vi "Martinas Aging Program v1.0c.vi"() -> ()   [LabVIEW 2011]
uses:
  <vilib>/ULx/Create Channel.llb/ULx Create Channel (DO-Digital Output).vi
  <vilib>/ULx/Write.llb/ULx Write (Digital U32 1Chan 1Samp).vi
  <instrlib>/Keithley 24XX/Keithley 24XX.lvlib
panel:
  out "Numeric":dbl
  out "Cell Settings Array":T1(array[cluster])=[{"Measure?"=TRUE, "Area (cm^2)"=0.0, "Cell Label"="", "Cell Description"="", "Time between scans (min)"=0.0, "Cell Position"=1, "Scan settings in queue"=0, "Sample holder"=1.0}, {"Measure?"=TRUE, "Area (cm^2)"=0.0, "Cell Label"="", "Cell Description"="", "Time between scans (min)"=0.0, "Cell Position"=2, "Scan settings in queue"=0, "Sample holder"=1.0}, {"Measure?"=TRUE, "Area (cm^2)"=0.0, "Cell Label"="", "Cell Description"="", "Time between scans (min)"=0.0, "Cell Position"=3, "Scan settings in queue"=0, "Sample holder"=1.0}, {"Measure?"=TRUE, "Area (cm^2)"=0.0, "Cell Label"="", "Cell Description"="", "Time between scans (min)"=0.0, "Cell Position"=4, "Scan settings in queue"=0, "Sample holder"=1.0}, {"Measure?"=TRUE, "Area (cm^2)"=0.0, "Cell Label"="", "Cell Description"="", "Time between scans (min)"=0.0, "Cell Position"=5, "Scan settings in queue"=0, "Sample holder"=1.0}, {"Measure?"=TRUE, "Area (cm^2)"=0.0, "Cell Label"="", "Cell Description"="", "Time between scans (min)"=0.0, "Cell Position"=6, "Scan settings in queue"=0, "Sample holder"=1.0}, {"Measure?"=TRUE, "Area (cm^2)"=0.0, "Cell Label"="", "Cell Description"="", "Time between scans (min)"=0.0, "Cell Position"=7, "Scan settings in queue"=0, "Sample holder"=1.0}, {"Measure?"=TRUE, "Area (cm^2)"=0.0, "Cell Label"="", "Cell Description"="", "Time between scans (min)"=0.0, "Cell Position"=8, "Scan settings in queue"=0, "Sample holder"=1.0}, {"Measure?"=TRUE, "Area (cm^2)"=0.0, "Cell Label"="", "Cell Description"="", "Time between scans (min)"=0.0, "Cell Position"=9, "Scan settings in queue"=0, "Sample holder"=1.0}, {"Measure?"=TRUE, "Area (cm^2)"=0.0, "Cell Label"="", "Cell Description"="", "Time between scans (min)"=0.0, "Cell Position"=10, "Scan settings in queue"=0, "Sample holder"=1.0}, {"Measure?"=TRUE, "Area (cm^2)"=0.0, "Cell Label"="", "Cell Description"="", "Time between scans (min)"=0.0, "Cell Position"=11, "Scan settings in queue"=0, "Sample holder"=1.0}, {"Measure?"=TRUE, "Area (cm^2)"=0.0, "Cell Label"="", "Cell Description"="", "Time between scans (min)"=0.0, "Cell Position"=12, "Scan settings in queue"=0, "Sample holder"=1.0}, {"Measure?"=TRUE, "Area (cm^2)"=0.0, "Cell Label"="", "Cell Description"="", "Time between scans (min)"=0.0, "Cell Position"=13, "Scan settings in queue"=0, "Sample holder"=1.0}, {"Measure?"=TRUE, "Area (cm^2)"=0.0, "Cell Label"="", "Cell Description"="", "Time between scans (min)"=0.0, "Cell Position"=14, "Scan settings in queue"=0, "Sample holder"=1.0}, {"Measure?"=TRUE, "Area (cm^2)"=0.0, "Cell Label"="", "Cell Description"="", "Time between scans (min)"=0.0, "Cell Position"=15, "Scan settings in queue"=0, "Sample holder"=1.0}, {"Measure?"=TRUE, "Area (cm^2)"=0.0, "Cell Label"="", "Cell Description"="", "Time between scans (min)"=0.0, "Cell Position"=16, "Scan settings in queue"=0, "Sample holder"=1.0}] {"Scan settings in queue" items=["Regular", "Inverted"]}
  in  "Port":refnum<k21>="Dev0/AuxPort"
  in  "VISA resource name":refnum<visa-resource-name>="GPIB0::24::INSTR"
  in  "Tab Control":T2(tab)
  in  "Cell Settings Array 1":T3(array[cluster])=[{"Measure?"=TRUE, "Area (cm^2)"=0.0, "Cell Label"="", "Cell Description"="", "Time between scans (s)"=0.0, "Cell Position"=1, "Scan settings in queue"=0, "Sample holder"=1.0}, {"Measure?"=TRUE, "Area (cm^2)"=0.0, "Cell Label"="", "Cell Description"="", "Time between scans (s)"=0.0, "Cell Position"=2, "Scan settings in queue"=0, "Sample holder"=1.0}, {"Measure?"=TRUE, "Area (cm^2)"=0.0, "Cell Label"="", "Cell Description"="", "Time between scans (s)"=0.0, "Cell Position"=3, "Scan settings in queue"=0, "Sample holder"=1.0}, {"Measure?"=TRUE, "Area (cm^2)"=0.0, "Cell Label"="", "Cell Description"="", "Time between scans (s)"=0.0, "Cell Position"=4, "Scan settings in queue"=0, "Sample holder"=1.0}, {"Measure?"=TRUE, "Area (cm^2)"=0.0, "Cell Label"="", "Cell Description"="", "Time between scans (s)"=0.0, "Cell Position"=5, "Scan settings in queue"=0, "Sample holder"=1.0}, {"Measure?"=TRUE, "Area (cm^2)"=0.0, "Cell Label"="", "Cell Description"="", "Time between scans (s)"=0.0, "Cell Position"=6, "Scan settings in queue"=0, "Sample holder"=1.0}, {"Measure?"=TRUE, "Area (cm^2)"=0.0, "Cell Label"="", "Cell Description"="", "Time between scans (s)"=0.0, "Cell Position"=7, "Scan settings in queue"=0, "Sample holder"=1.0}, {"Measure?"=TRUE, "Area (cm^2)"=0.0, "Cell Label"="", "Cell Description"="", "Time between scans (s)"=0.0, "Cell Position"=8, "Scan settings in queue"=0, "Sample holder"=1.0}, {"Measure?"=TRUE, "Area (cm^2)"=0.0, "Cell Label"="", "Cell Description"="", "Time between scans (s)"=0.0, "Cell Position"=9, "Scan settings in queue"=0, "Sample holder"=1.0}, {"Measure?"=TRUE, "Area (cm^2)"=0.0, "Cell Label"="", "Cell Description"="", "Time between scans (s)"=0.0, "Cell Position"=10, "Scan settings in queue"=0, "Sample holder"=1.0}, {"Measure?"=TRUE, "Area (cm^2)"=0.0, "Cell Label"="", "Cell Description"="", "Time between scans (s)"=0.0, "Cell Position"=11, "Scan settings in queue"=0, "Sample holder"=1.0}, {"Measure?"=TRUE, "Area (cm^2)"=0.0, "Cell Label"="", "Cell Description"="", "Time between scans (s)"=0.0, "Cell Position"=12, "Scan settings in queue"=0, "Sample holder"=1.0}, {"Measure?"=TRUE, "Area (cm^2)"=0.0, "Cell Label"="", "Cell Description"="", "Time between scans (s)"=0.0, "Cell Position"=13, "Scan settings in queue"=0, "Sample holder"=1.0}, {"Measure?"=TRUE, "Area (cm^2)"=0.0, "Cell Label"="", "Cell Description"="", "Time between scans (s)"=0.0, "Cell Position"=14, "Scan settings in queue"=0, "Sample holder"=1.0}, {"Measure?"=TRUE, "Area (cm^2)"=0.0, "Cell Label"="", "Cell Description"="", "Time between scans (s)"=0.0, "Cell Position"=15, "Scan settings in queue"=0, "Sample holder"=1.0}, {"Measure?"=TRUE, "Area (cm^2)"=0.0, "Cell Label"="", "Cell Description"="", "Time between scans (s)"=0.0, "Cell Position"=16, "Scan settings in queue"=0, "Sample holder"=1.0}] {"Scan settings in queue" items=["Regular", "Inverted", "Test"]}
  in  "Upload from Spreadsheet?":bool
  in  "Upload Spreadsheet path":path
  in  "Save to Spreadsheet?":bool
  in  "Save Spreadsheet Path":path
  in  "Cell Settings Array 2":T1(array[cluster])=[{"Measure?"=TRUE, "Area (cm^2)"=0.0, "Cell Label"="", "Cell Description"="", "Time between scans (min)"=0.0, "Cell Position"=1, "Scan settings in queue"=0, "Sample holder"=2.0}, {"Measure?"=TRUE, "Area (cm^2)"=0.0, "Cell Label"="", "Cell Description"="", "Time between scans (min)"=0.0, "Cell Position"=2, "Scan settings in queue"=0, "Sample holder"=2.0}, {"Measure?"=TRUE, "Area (cm^2)"=0.0, "Cell Label"="", "Cell Description"="", "Time between scans (min)"=0.0, "Cell Position"=3, "Scan settings in queue"=0, "Sample holder"=2.0}, {"Measure?"=TRUE, "Area (cm^2)"=0.0, "Cell Label"="", "Cell Description"="", "Time between scans (min)"=0.0, "Cell Position"=4, "Scan settings in queue"=0, "Sample holder"=2.0}, {"Measure?"=TRUE, "Area (cm^2)"=0.0, "Cell Label"="", "Cell Description"="", "Time between scans (min)"=0.0, "Cell Position"=5, "Scan settings in queue"=0, "Sample holder"=2.0}, {"Measure?"=TRUE, "Area (cm^2)"=0.0, "Cell Label"="", "Cell Description"="", "Time between scans (min)"=0.0, "Cell Position"=6, "Scan settings in queue"=0, "Sample holder"=2.0}, {"Measure?"=TRUE, "Area (cm^2)"=0.0, "Cell Label"="", "Cell Description"="", "Time between scans (min)"=0.0, "Cell Position"=7, "Scan settings in queue"=0, "Sample holder"=2.0}, {"Measure?"=TRUE, "Area (cm^2)"=0.0, "Cell Label"="", "Cell Description"="", "Time between scans (min)"=0.0, "Cell Position"=8, "Scan settings in queue"=0, "Sample holder"=2.0}, {"Measure?"=TRUE, "Area (cm^2)"=0.0, "Cell Label"="", "Cell Description"="", "Time between scans (min)"=0.0, "Cell Position"=9, "Scan settings in queue"=0, "Sample holder"=2.0}, {"Measure?"=TRUE, "Area (cm^2)"=0.0, "Cell Label"="", "Cell Description"="", "Time between scans (min)"=0.0, "Cell Position"=10, "Scan settings in queue"=0, "Sample holder"=2.0}, {"Measure?"=TRUE, "Area (cm^2)"=0.0, "Cell Label"="", "Cell Description"="", "Time between scans (min)"=0.0, "Cell Position"=11, "Scan settings in queue"=0, "Sample holder"=2.0}, {"Measure?"=TRUE, "Area (cm^2)"=0.0, "Cell Label"="", "Cell Description"="", "Time between scans (min)"=0.0, "Cell Position"=12, "Scan settings in queue"=0, "Sample holder"=2.0}, {"Measure?"=TRUE, "Area (cm^2)"=0.0, "Cell Label"="", "Cell Description"="", "Time between scans (min)"=0.0, "Cell Position"=13, "Scan settings in queue"=0, "Sample holder"=2.0}, {"Measure?"=TRUE, "Area (cm^2)"=0.0, "Cell Label"="", "Cell Description"="", "Time between scans (min)"=0.0, "Cell Position"=14, "Scan settings in queue"=0, "Sample holder"=2.0}, {"Measure?"=TRUE, "Area (cm^2)"=0.0, "Cell Label"="", "Cell Description"="", "Time between scans (min)"=0.0, "Cell Position"=15, "Scan settings in queue"=0, "Sample holder"=2.0}, {"Measure?"=TRUE, "Area (cm^2)"=0.0, "Cell Label"="", "Cell Description"="", "Time between scans (min)"=0.0, "Cell Position"=16, "Scan settings in queue"=0, "Sample holder"=2.0}] {"Scan settings in queue" items=["Regular", "Inverted", "Test"]}
  in  "Upload Spreadsheet path 2":path
  in  "Upload from Spreadsheet? 2":bool
  in  "Save Spreadsheet Path 2":path
  in  "Save to Spreadsheet?  2":bool
  in  "Cell Settings Array 3":T1(array[cluster])=[{"Measure?"=TRUE, "Area (cm^2)"=0.0, "Cell Label"="", "Cell Description"="", "Time between scans (min)"=0.0, "Cell Position"=1, "Scan settings in queue"=0, "Sample holder"=3.0}, {"Measure?"=TRUE, "Area (cm^2)"=0.0, "Cell Label"="", "Cell Description"="", "Time between scans (min)"=0.0, "Cell Position"=2, "Scan settings in queue"=0, "Sample holder"=3.0}, {"Measure?"=TRUE, "Area (cm^2)"=0.0, "Cell Label"="", "Cell Description"="", "Time between scans (min)"=0.0, "Cell Position"=3, "Scan settings in queue"=0, "Sample holder"=3.0}, {"Measure?"=TRUE, "Area (cm^2)"=0.0, "Cell Label"="", "Cell Description"="", "Time between scans (min)"=0.0, "Cell Position"=4, "Scan settings in queue"=0, "Sample holder"=3.0}, {"Measure?"=TRUE, "Area (cm^2)"=0.0, "Cell Label"="", "Cell Description"="", "Time between scans (min)"=0.0, "Cell Position"=5, "Scan settings in queue"=0, "Sample holder"=3.0}, {"Measure?"=TRUE, "Area (cm^2)"=0.0, "Cell Label"="", "Cell Description"="", "Time between scans (min)"=0.0, "Cell Position"=6, "Scan settings in queue"=0, "Sample holder"=3.0}, {"Measure?"=TRUE, "Area (cm^2)"=0.0, "Cell Label"="", "Cell Description"="", "Time between scans (min)"=0.0, "Cell Position"=7, "Scan settings in queue"=0, "Sample holder"=3.0}, {"Measure?"=TRUE, "Area (cm^2)"=0.0, "Cell Label"="", "Cell Description"="", "Time between scans (min)"=0.0, "Cell Position"=8, "Scan settings in queue"=0, "Sample holder"=3.0}, {"Measure?"=TRUE, "Area (cm^2)"=0.0, "Cell Label"="", "Cell Description"="", "Time between scans (min)"=0.0, "Cell Position"=9, "Scan settings in queue"=0, "Sample holder"=3.0}, {"Measure?"=TRUE, "Area (cm^2)"=0.0, "Cell Label"="", "Cell Description"="", "Time between scans (min)"=0.0, "Cell Position"=10, "Scan settings in queue"=0, "Sample holder"=3.0}, {"Measure?"=TRUE, "Area (cm^2)"=0.0, "Cell Label"="", "Cell Description"="", "Time between scans (min)"=0.0, "Cell Position"=11, "Scan settings in queue"=0, "Sample holder"=3.0}, {"Measure?"=TRUE, "Area (cm^2)"=0.0, "Cell Label"="", "Cell Description"="", "Time between scans (min)"=0.0, "Cell Position"=12, "Scan settings in queue"=0, "Sample holder"=3.0}, {"Measure?"=TRUE, "Area (cm^2)"=0.0, "Cell Label"="", "Cell Description"="", "Time between scans (min)"=0.0, "Cell Position"=13, "Scan settings in queue"=0, "Sample holder"=3.0}, {"Measure?"=TRUE, "Area (cm^2)"=0.0, "Cell Label"="", "Cell Description"="", "Time between scans (min)"=0.0, "Cell Position"=14, "Scan settings in queue"=0, "Sample holder"=3.0}, {"Measure?"=TRUE, "Area (cm^2)"=0.0, "Cell Label"="", "Cell Description"="", "Time between scans (min)"=0.0, "Cell Position"=15, "Scan settings in queue"=0, "Sample holder"=3.0}, {"Measure?"=TRUE, "Area (cm^2)"=0.0, "Cell Label"="", "Cell Description"="", "Time between scans (min)"=0.0, "Cell Position"=16, "Scan settings in queue"=0, "Sample holder"=3.0}] {"Scan settings in queue" items=["Regular", "Inverted", "Test"]}
  in  "Upload Spreadsheet path 3":path
  in  "Upload from Spreadsheet? 3":bool
  in  "Save Spreadsheet Path 3":path
  in  "Save to Spreadsheet?  3":bool
  in  "Cell Settings Array 4":T1(array[cluster])=[{"Measure?"=TRUE, "Area (cm^2)"=0.0, "Cell Label"="", "Cell Description"="", "Time between scans (min)"=0.0, "Cell Position"=1, "Scan settings in queue"=0, "Sample holder"=4.0}, {"Measure?"=TRUE, "Area (cm^2)"=0.0, "Cell Label"="", "Cell Description"="", "Time between scans (min)"=0.0, "Cell Position"=2, "Scan settings in queue"=0, "Sample holder"=4.0}, {"Measure?"=TRUE, "Area (cm^2)"=0.0, "Cell Label"="", "Cell Description"="", "Time between scans (min)"=0.0, "Cell Position"=3, "Scan settings in queue"=0, "Sample holder"=4.0}, {"Measure?"=TRUE, "Area (cm^2)"=0.0, "Cell Label"="", "Cell Description"="", "Time between scans (min)"=0.0, "Cell Position"=4, "Scan settings in queue"=0, "Sample holder"=4.0}, {"Measure?"=TRUE, "Area (cm^2)"=0.0, "Cell Label"="", "Cell Description"="", "Time between scans (min)"=0.0, "Cell Position"=5, "Scan settings in queue"=0, "Sample holder"=4.0}, {"Measure?"=TRUE, "Area (cm^2)"=0.0, "Cell Label"="", "Cell Description"="", "Time between scans (min)"=0.0, "Cell Position"=6, "Scan settings in queue"=0, "Sample holder"=4.0}, {"Measure?"=TRUE, "Area (cm^2)"=0.0, "Cell Label"="", "Cell Description"="", "Time between scans (min)"=0.0, "Cell Position"=7, "Scan settings in queue"=0, "Sample holder"=4.0}, {"Measure?"=TRUE, "Area (cm^2)"=0.0, "Cell Label"="", "Cell Description"="", "Time between scans (min)"=0.0, "Cell Position"=8, "Scan settings in queue"=0, "Sample holder"=4.0}, {"Measure?"=TRUE, "Area (cm^2)"=0.0, "Cell Label"="", "Cell Description"="", "Time between scans (min)"=0.0, "Cell Position"=9, "Scan settings in queue"=0, "Sample holder"=4.0}, {"Measure?"=TRUE, "Area (cm^2)"=0.0, "Cell Label"="", "Cell Description"="", "Time between scans (min)"=0.0, "Cell Position"=10, "Scan settings in queue"=0, "Sample holder"=4.0}, {"Measure?"=TRUE, "Area (cm^2)"=0.0, "Cell Label"="", "Cell Description"="", "Time between scans (min)"=0.0, "Cell Position"=11, "Scan settings in queue"=0, "Sample holder"=4.0}, {"Measure?"=TRUE, "Area (cm^2)"=0.0, "Cell Label"="", "Cell Description"="", "Time between scans (min)"=0.0, "Cell Position"=12, "Scan settings in queue"=0, "Sample holder"=4.0}, {"Measure?"=TRUE, "Area (cm^2)"=0.0, "Cell Label"="", "Cell Description"="", "Time between scans (min)"=0.0, "Cell Position"=13, "Scan settings in queue"=0, "Sample holder"=4.0}, {"Measure?"=TRUE, "Area (cm^2)"=0.0, "Cell Label"="", "Cell Description"="", "Time between scans (min)"=0.0, "Cell Position"=14, "Scan settings in queue"=0, "Sample holder"=4.0}, {"Measure?"=TRUE, "Area (cm^2)"=0.0, "Cell Label"="", "Cell Description"="", "Time between scans (min)"=0.0, "Cell Position"=15, "Scan settings in queue"=0, "Sample holder"=4.0}, {"Measure?"=TRUE, "Area (cm^2)"=0.0, "Cell Label"="", "Cell Description"="", "Time between scans (min)"=0.0, "Cell Position"=16, "Scan settings in queue"=0, "Sample holder"=4.0}] {"Scan settings in queue" items=["Regular", "Inverted", "Test"]}
  in  "Upload Spreadsheet path 4":path
  in  "Upload from Spreadsheet? 4":bool
  in  "Save Spreadsheet Path 4":path
  in  "Save to Spreadsheet?  4":bool
  in  "Stop Scan":bool
  in  "Start Scan":bool
  out "Table":string[][](table)
  out "JV Curve":cluster{"Y":dbl[], "Y":dbl[]}[](graph)
  in  "Upload to the Queue":bool
  in  "Stop Labview":bool
  in  "Scan settings":u16(ring) items=["Regular", "Inverted", "Test"]
  in  "Scan Settings JV":T4={"Light Intensity (Suns)"=1.0, "Stabilization Time (s)"=5.0, "Maximum Voltage (V)"=0.0, "Minimum Voltage (V)"=-1.0, "Range Options"=0, "Scan Direction\nDU (T), UD (F)"=TRUE, "Step Size (V)"=0.01, "Source Delay (s)"=0.15} {"Range Options" items=["Auto Range", "Semi-Auto Range", "100 uA", "1 mA", "10 mA", "100 mA", "1A"]}
  in  "Scan Setting Name":string
  in  "Add to Menu ring":bool
  out "Show me Scan \nSettings JV set":T4={"Light Intensity (Suns)"=1.0, "Stabilization Time (s)"=5.0, "Maximum Voltage (V)"=0.0, "Minimum Voltage (V)"=-1.0, "Range Options"=0, "Scan Direction\nDU (T), UD (F)"=TRUE, "Step Size (V)"=0.01, "Source Delay (s)"=0.15} {"Range Options" items=["Auto Range", "Semi-Auto Range", "100 uA", "1 mA", "10 mA", "100 mA", "1A"]}
  in  "Delete from Menu Ring":bool
  in  "Queue":T5(array[cluster]) {"Scan settings in queue" items=["Regular", "Inverted", "Test"]; "Time of the last scan (s)" format="%<%H:%M:%S>t"; "When did you stick it in?" format="%<%H:%M:%S>t"; "Time to next scan (s)" format="%<%H:%M:%S>t"; "Time in rig (s)" format="%<%H:%M:%S>t"}
  out "TIMER":dbl format="%<%H:%M:%S>t"
  out "Username":string caption="Logged in as:"
  # "Cell Ageing Routine"
  # "Time between Scans (s)"
  # "Cell\nPosition"
  # "Sample\nHolder"
  # "On = working cell\nOff = not working cell"
  # "Area"
  # "Label"
  # "Comment"
  # "Scan Settings"
  # "Time between Scans (s)"
  # "Cell\nPosition"
  # "Sample\nHolder"
  # "On = working cell\nOff = not working cell"
  # "Area"
  # "Label"
  # "Comment"
  # "Scan Settings"
  # "Time between Scans (s)"
  # "Cell\nPosition"
  # "Sample\nHolder"
  # "On = working cell\nOff = not working cell"
  # "Area"
  # "Label"
  # "Comment"
  # "Scan Settings"
  # "Time between Scans (s)"
  # "Cell\nPosition"
  # "Sample\nHolder"
  # "On = working cell\nOff = not working cell"
  # "Area"
  # "Label"
  # "Comment"
  # "Scan Settings"
  # "Area\n(cm^2)"
  # "Scan\nwait(s)"
  # "Cell \nposition"
  # "Time in rig\n(hrs)"
  # "Time since last scan (hrs)"
  # "Scan\nnumber"
  # "Time\nZero"
  # "Time of \nlast scan"
  # "Sample\nHolder"
  # "On = working\nOff = not working"
  # "Label"
  # "Comment"
  # "Scan Settings"
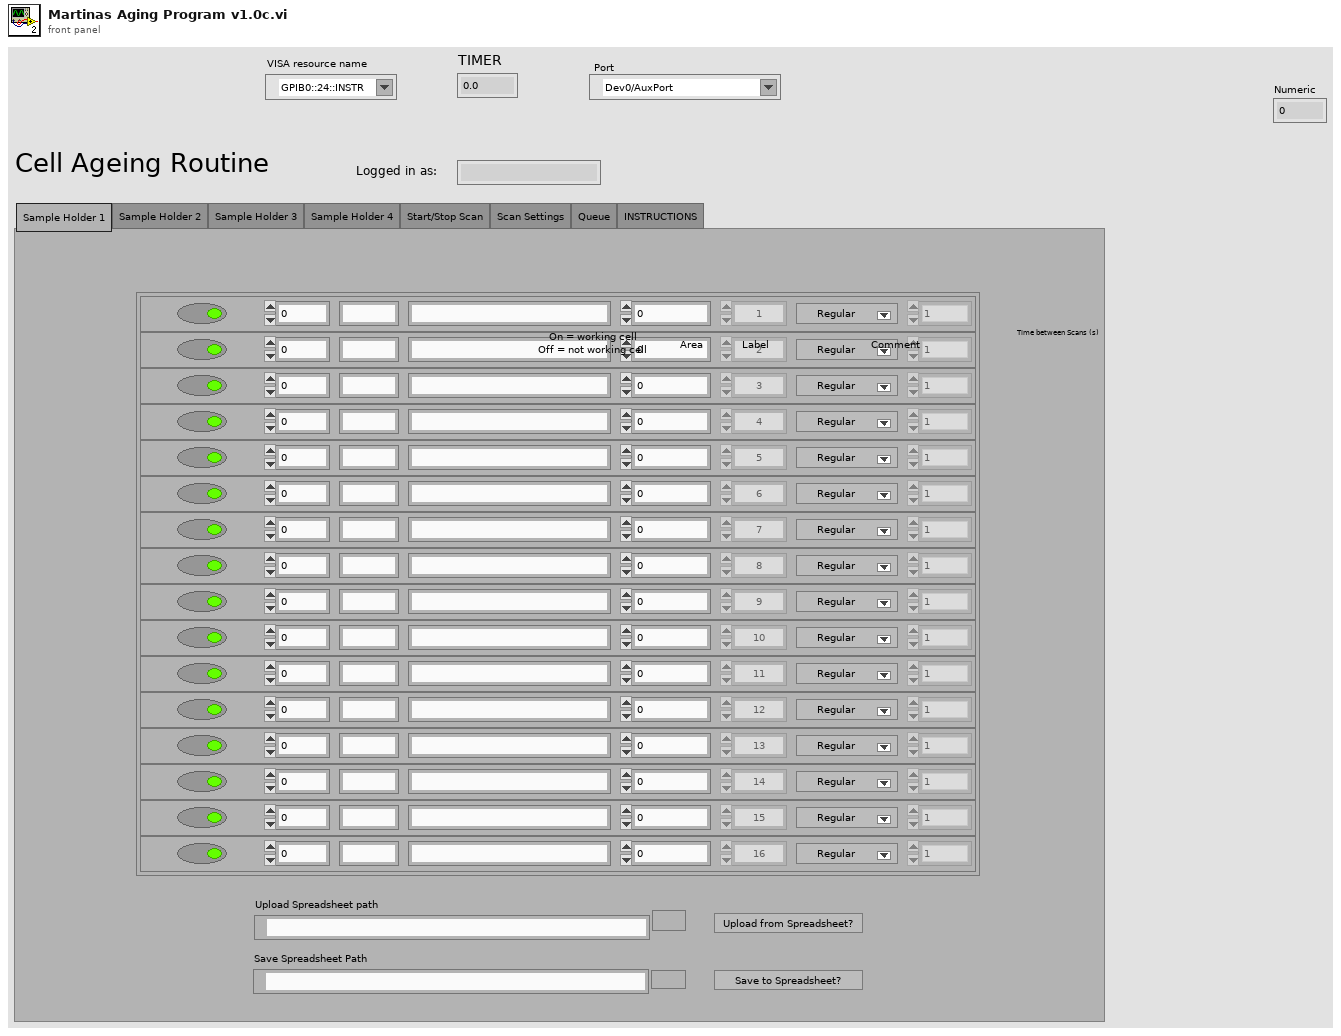
[diagram p1: front panel]
types:
  T1 = cluster{"Measure?":bool, "Area (cm^2)":dbl, "Cell Label":string, "Cell Description":string, "Time between scans (min)":dbl, "Cell Position":i32, "Scan settings in queue":u16, "Sample holder":dbl}[]
  T2 = enum32{"Sample Holder 1", "Sample Holder 2", "Sample Holder 3", "Sample Holder 4", "Start/Stop Scan", "Scan Settings", "Queue", "INSTRUCTIONS"}
  T3 = cluster{"Measure?":bool, "Area (cm^2)":dbl, "Cell Label":string, "Cell Description":string, "Time between scans (s)":dbl, "Cell Position":i32, "Scan settings in queue":u16, "Sample holder":dbl}[]
  T4 = cluster{"Light Intensity (Suns)":dbl, "Stabilization Time (s)":dbl, "Maximum Voltage (V)":dbl, "Minimum Voltage (V)":dbl, "Range Options":u16, "Scan Direction\nDU (T), UD (F)":bool, "Step Size (V)":dbl, "Source Delay (s)":dbl}
  T5 = cluster{"Measure?":bool, "Area (cm^2)":dbl, "Cell Label":string, "Cell Description":string, "Cell Position":i32, "Time in rig (s)":dbl, "Time to next scan (s)":dbl, "Scan number":dbl, "When did you stick it in?":dbl, "Time between scans (s)":dbl, "Time of the last scan (s)":dbl, "Scan settings in queue":u16, "Sample Holder":dbl}[]
  T6 = enum8{"Enabled", "Disabled", "Disabled and Grayed Out"}
  T7 = cluster{"Light Intensity (Suns)":dbl, "Stabilization Time (s)":dbl, "Maximum Voltage (V)":dbl, "Minimum Voltage (V)":dbl, "Range Options":u16, "Scan Direction\nDU (T), UD (F)":bool, "Step Size (V)":dbl, "Source Delay (s)":dbl}[]
  T8 = cluster{"Measure?":bool, "Area (cm^2)":dbl, "Cell Label":string, "Cell Description":string, "Cell Position":i32, "Time in rig (s)":dbl, "Time to next scan (s)":dbl, "Scan number":dbl, "When did you stick it in?":dbl, "Time between scans (s)":dbl, "Time of the last scan (s)":dbl, "Scan settings in queue":u16, "Sample Holder":dbl}
  T9 = typedef "imagedata.ctl" = cluster{"image type":i32, "image depth":i32, "image":u8[], "mask":u8[], "colors":u32[], "Rectangle":cluster{"left":i16, "top":i16, "right":i16, "bottom":i16}}
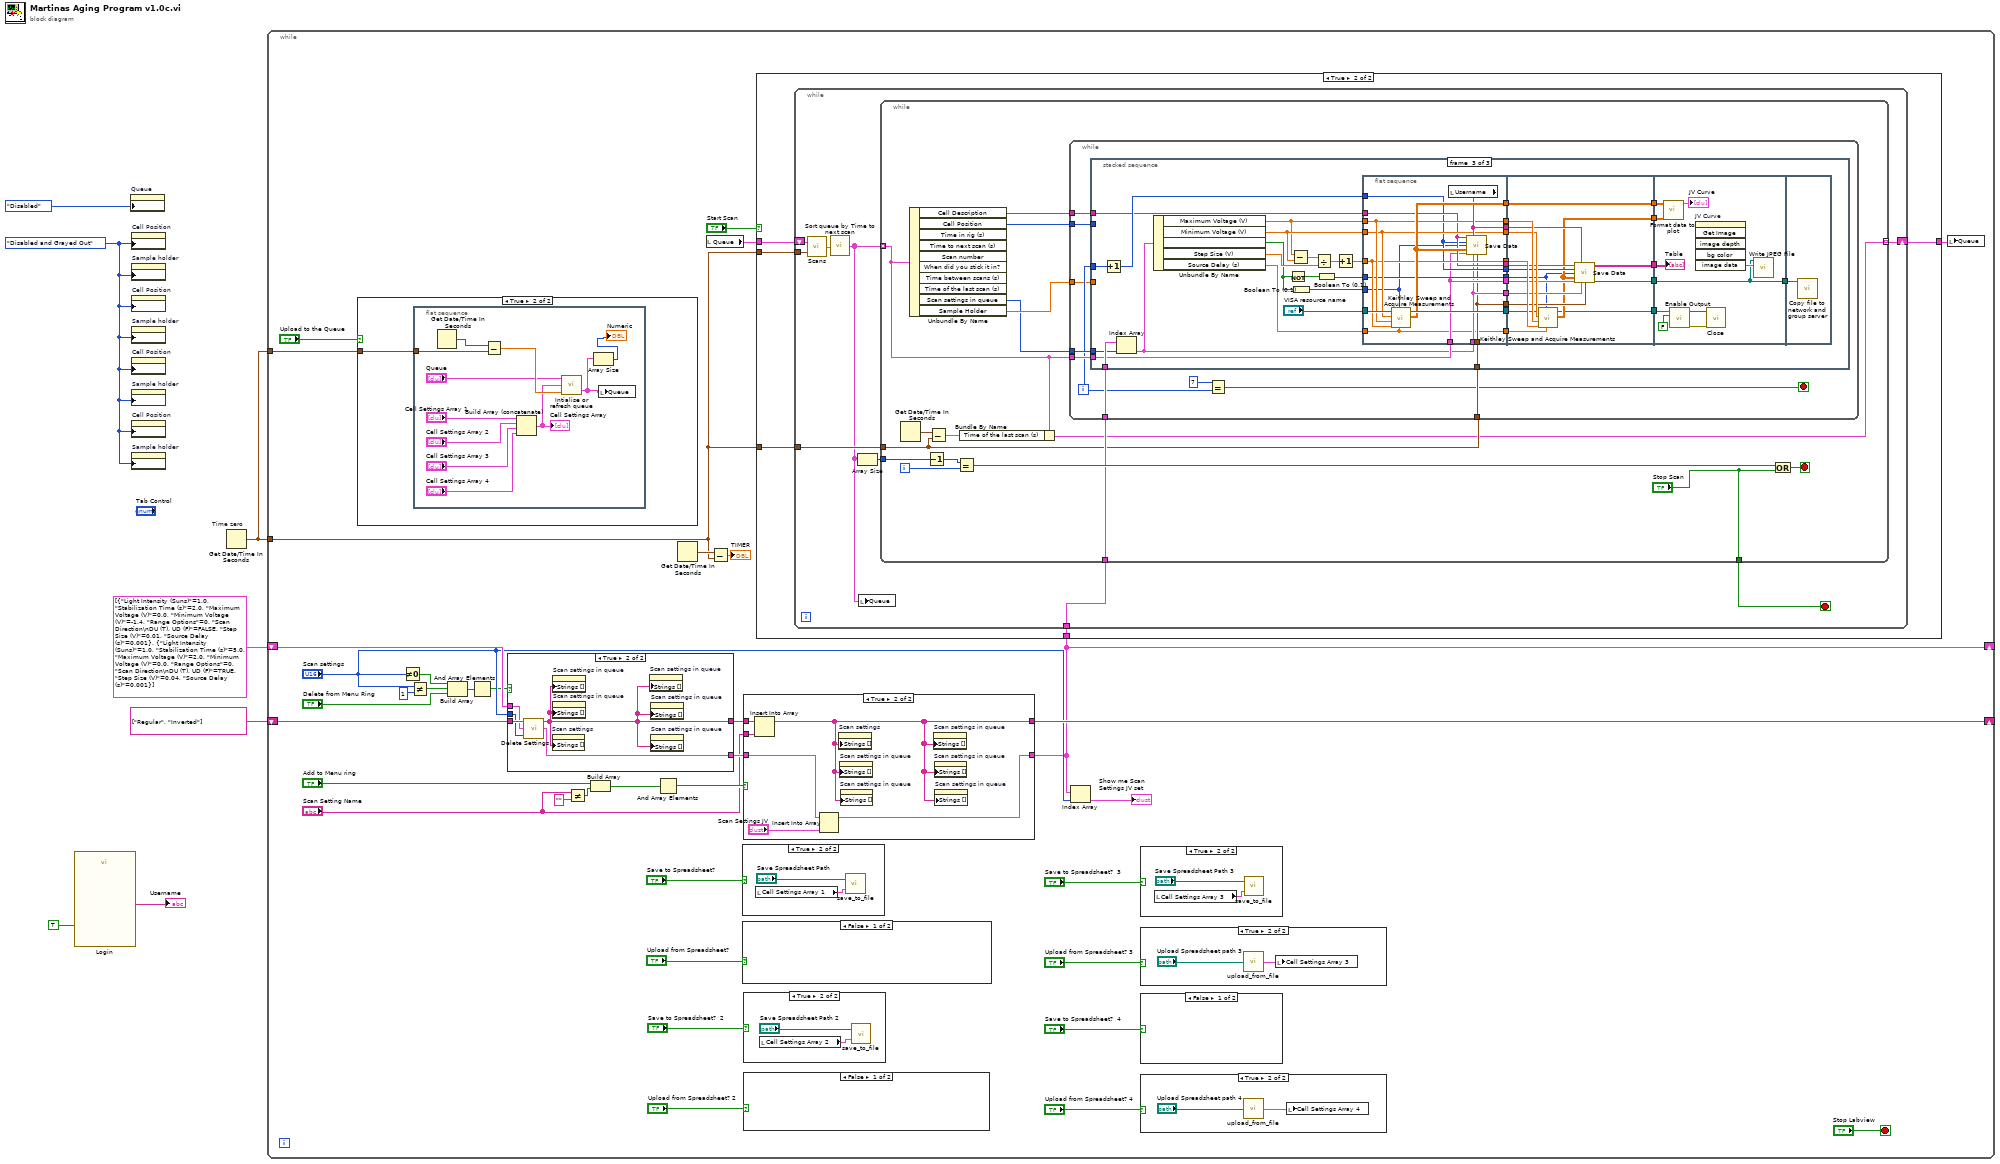
[diagram p0: block diagram]
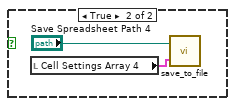
[diagram p2: hidden frame]
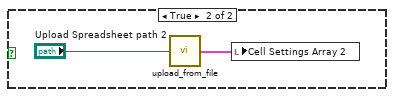
[diagram p7: hidden frame]
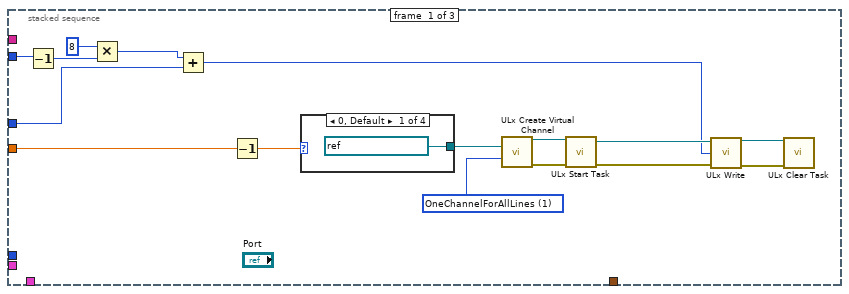
[diagram p9: hidden frame]
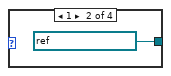
[diagram p10: hidden frame]
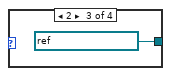
[diagram p11: hidden frame]
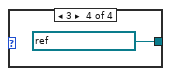
[diagram p12: hidden frame]
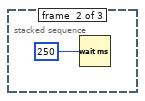
[diagram p13: hidden frame]
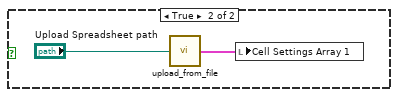
[diagram p18: hidden frame]
diagram:
  w4 = T6."Disabled and Grayed Out" ("Disabled")
  n1 = call "Login"("Enable"=TRUE) -> ("Username"=→"Username":string)  [unwired: 16 in, 2 out]
  n2 = property on="Queue" class="Arr (strict)"("DisabledEnum"=T6."Disabled" ("Disabled")) -> ()  [unwired: 2 in, 2 out]
  n3 = property on="Cell Position" class="DigNum (strict)"("DisabledEnum"=w4) -> ()  [unwired: 2 in, 2 out]
  n4 = property on="Sample holder" class="DigNum (strict)"("DisabledEnum"=w4) -> ()  [unwired: 2 in, 2 out]
  n5 = property on="Cell Position" class="DigNum (strict)"("DisabledEnum"=w4) -> ()  [unwired: 2 in, 2 out]
  n6 = property on="Sample holder" class="DigNum (strict)"("DisabledEnum"=w4) -> ()  [unwired: 2 in, 2 out]
  n7 = property on="Cell Position" class="DigNum (strict)"("DisabledEnum"=w4) -> ()  [unwired: 2 in, 2 out]
  n8 = property on="Sample holder" class="DigNum (strict)"("DisabledEnum"=w4) -> ()  [unwired: 2 in, 2 out]
  n9 = property on="Cell Position" class="DigNum (strict)"("DisabledEnum"=w4) -> ()  [unwired: 2 in, 2 out]
  n10 = property on="Sample holder" class="DigNum (strict)"("DisabledEnum"=w4) -> ()  [unwired: 2 in, 2 out]
  n11 = Get Date/Time In Seconds "Time zero"() -> (seconds since 1Jan1904=w5:timestamp)
  n12 = while {
    tunnel: w5 -> [w41]
    shift-right: [w11] -> _
    shift-left: T7 [{"Light Intensity (Suns)"=1.0, "Stabilization Time (s)"=2.0, "Maximum Voltage (V)"=0.0, "Minimum Voltage (V)"=-1.4, "Range Options"=0, "Scan Direction\nDU (T), UD (F)"=FALSE, "Step Size (V)"=0.01, "Source Delay (s)"=0.001}, {"Light Intensity (Suns)"=1.0, "Stabilization Time (s)"=5.0, "Maximum Voltage (V)"=2.0, "Minimum Voltage (V)"=0.0, "Range Options"=0, "Scan Direction\nDU (T), UD (F)"=TRUE, "Step Size (V)"=0.04, "Source Delay (s)"=0.001}] ("JV curve scan settings 2") -> [w37]
    shift-right: [w40] -> _
    shift-left: string[] ["Regular", "Inverted"] ("Strings []") -> [w38]
    tunnel: w5 -> [w10]
    stop <- "Stop Labview" stop-if-true
    n13 = case shown="True" "Upload to the Queue" {
      tunnel: w41 -> [_ w216]
      frame False {
      }
      frame True {
        n14 = flat-sequence {
          tunnel: w216 -> [w227]
          frame #0 {
            n15 = Get Date/Time In Seconds() -> (seconds since 1Jan1904=w226:timestamp)
            n16 = Subtract(x=w226, y=w227) -> (x-y=w225:dbl)
            n17 = Build Array (concatenate)("Cell Settings Array 1", "Cell Settings Array 2", "Cell Settings Array 3", "Cell Settings Array 4") -> (w219:T1)
            "Cell Settings Array" <- w219
            n18 = call "Intialise or refresh queue.vi"("When did you stick it in?"=w225, "Cell Settings Array"=w219, "Queue in"="Queue") -> ("Queue out"=w218:T5)  [unwired: 1 in]
            n19 = Array Size(array=w218) -> (size(s)=→"Numeric":i32)
            n20 = local write "Queue"(w218) -> ()
          }
        }
      }
    }
    n21 = Not Equal To 0?(x="Scan settings") -> (x != 0?=w34:bool)
    n22 = Not Equal?(x="Scan settings", y=u16 1) -> (x != y?=w31:bool)
    n23 = Build Array(w34, w31, "Delete from Menu Ring") -> (w29:bool[])
    n24 = And Array Elements(Boolean array=w29) -> (logical AND=w28:bool)
    n25 = case shown="True" w28 {
      tunnel: w38 -> [w201 w207]
      tunnel: w37 -> [w202 w206]
      tunnel: "Scan settings" -> [_ w205]
      tunnel: [w201 w203] -> w36
      tunnel: [w202 w204] -> w35
      frame False {
      }
      frame True {
        n26 = call "Delete Settings.vi"("Scan settings"=w205, "JV curve scan settings"=w206, "Strings In"=w207) -> ("JV curve scan settings Out"=w204:T7, "Strings Out"=w203:string[])  [unwired: 1 out]
        n27 = property on="Scan settings" class="Ring (strict)"("Strings []"=w203) -> ()  [unwired: 2 in, 2 out]
        n28 = property on="Scan settings in queue" class="Ring (strict)"("Strings []"=w203) -> ()  [unwired: 2 in, 2 out]
        n29 = property on="Scan settings in queue" class="Ring (strict)"("Strings []"=w203) -> ()  [unwired: 2 in, 2 out]
        n30 = property on="Scan settings in queue" class="Ring (strict)"("Strings []"=w203) -> ()  [unwired: 2 in, 2 out]
        n31 = property on="Scan settings in queue" class="Ring (strict)"("Strings []"=w203) -> ()  [unwired: 2 in, 2 out]
        n32 = property on="Scan settings in queue" class="Ring (strict)"("Strings []"=w203) -> ()  [unwired: 2 in, 2 out]
      }
    }
    n33 = Not Equal?(x="Scan Setting Name", y="") -> (x != y?=w25:bool)
    n34 = Build Array("Add to Menu ring", w25) -> (w26:bool[])
    n35 = And Array Elements(Boolean array=w26) -> (logical AND=w23:bool)
    n36 = Get Date/Time In Seconds() -> (seconds since 1Jan1904=w20:timestamp)
    n37 = local read "Queue"() -> (w19:T5)
    n38 = Subtract(x=w20, y=w10) -> (x-y=→"TIMER":dbl)
    n39 = case shown="True" "Save to Spreadsheet?" {
      frame False {
      }
      frame True {
        n40 = local read "Cell Settings Array 1"() -> (w228:T3)
        n41 = call "save_to_file.vi"("Cell Settings Array 4"=w228, "Save Path"="Save Spreadsheet Path") -> ()  [unwired: 1 in]
      }
    }
    n42 = case shown="False" "Upload from Spreadsheet?" {
      frame False {
      }
      frame True {
        n43 = call "upload_from_file.vi"("Spreadsheet path"="Upload Spreadsheet path") -> ("Cell Settings Array 4"=w230:T1)
        n44 = local write "Cell Settings Array 1"(w230) -> ()
      }
    }
    n45 = case shown="True" w23 {
      tunnel: w35 -> [w209 w215]
      tunnel: [w209 w214] -> w11
      tunnel: w36 -> [w208 w212]
      tunnel: [w208 w210] -> w40
      tunnel: "Scan Setting Name" -> [_ w211]
      frame False {
      }
      frame True {
        n46 = Insert Into Array(array=w212, new element=w211) -> (w210:string[])  [unwired: 1 in]
        n47 = Insert Into Array(array=w215, new element="Scan Settings JV") -> (w214:T7)  [unwired: 1 in]
        n48 = property on="Scan settings" class="Ring (strict)"("Strings []"=w210) -> ()  [unwired: 2 in, 2 out]
        n49 = property on="Scan settings in queue" class="Ring (strict)"("Strings []"=w210) -> ()  [unwired: 2 in, 2 out]
        n50 = property on="Scan settings in queue" class="Ring (strict)"("Strings []"=w210) -> ()  [unwired: 2 in, 2 out]
        n51 = property on="Scan settings in queue" class="Ring (strict)"("Strings []"=w210) -> ()  [unwired: 2 in, 2 out]
        n52 = property on="Scan settings in queue" class="Ring (strict)"("Strings []"=w210) -> ()  [unwired: 2 in, 2 out]
        n53 = property on="Scan settings in queue" class="Ring (strict)"("Strings []"=w210) -> ()  [unwired: 2 in, 2 out]
      }
    }
    n54 = case shown="True" "Save to Spreadsheet?  2" {
      frame False {
      }
      frame True {
        n55 = local read "Cell Settings Array 2"() -> (w53:T1)
        n56 = call "save_to_file.vi"("Cell Settings Array 4"=w53, "Save Path"="Save Spreadsheet Path 2") -> ()  [unwired: 1 in]
      }
    }
    n57 = case shown="False" "Upload from Spreadsheet? 2" {
      frame False {
      }
      frame True {
        n58 = call "upload_from_file.vi"("Spreadsheet path"="Upload Spreadsheet path 2") -> ("Cell Settings Array 4"=w55:T1)
        n59 = local write "Cell Settings Array 2"(w55) -> ()
      }
    }
    n60 = case shown="True" "Start Scan" {
      tunnel: w19 -> [w57 w62]
      tunnel: w10 -> [_ w61]
      tunnel: [w57 w59] -> w9
      tunnel: w11 -> [_ w60]
      tunnel: w10 -> [_ w58]
      frame False {
      }
      frame True {
        n61 = while {
          tunnel: w61 -> [w70]
          tunnel: w60 -> [w68]
          shift-right: [w66] -> w59
          shift-left: w62 -> [w71]
          tunnel: w58 -> [w65]
          stop <- w63 stop-if-true
          n62 = call "Scans.vi"("Time zero (sec)"=w70, "Queue in"=w71) -> ("Queue out"=w69:T5)
          n63 = call "Sort queue by Time to next scan.vi"("Queue"=w69) -> ("Queue Out"=w64:T5)  [unwired: 4 in]
          n64 = Array Size(array=w64) -> (size(s)=w67:i32)
          n65 = local write "Queue"(w64) -> ()
          n66 = while {
            tunnel: w64 -> [w76] mode=indexing
            tunnel: w68 -> [w75]
            tunnel: w67 -> [w85]
            tunnel: [w73] -> w66 mode=indexing
            tunnel: w65 -> [w74]
            tunnel: ["Stop Scan"] -> w63
            i -> [w87]
            stop <- w84 stop-if-true
            n67 = Get Date/Time In Seconds() -> (seconds since 1Jan1904=w83:timestamp)
            n68 = Unbundle By Name(w76) -> ("Cell Description"=w80:string, "Cell Position"=w79:i32, "Scan settings in queue"=w77:u16, "Sample Holder"=w78:dbl)  [unwired: 6 out]
            n69 = Decrement(x=w85) -> (x-1=w86:i32)
            n70 = Subtract(x=w83, y=w74) -> (x-y=w82:dbl)
            n71 = Equal?(x=w86, y=w87) -> (x = y?=w81:bool)
            n72 = Bundle By Name(cluster=w76, "Time of the last scan (s)"=w82) -> (w73:T8)
            n73 = while {
              tunnel: w75 -> [w97]
              tunnel: w77 -> [w96]
              tunnel: w76 -> [w95]
              tunnel: w79 -> [w94]
              tunnel: w78 -> [w91]
              tunnel: w80 -> [w90]
              tunnel: w74 -> [w89]
              i -> [w92]
              stop <- w88 stop-if-true
              n74 = stacked-sequence {
                tunnel: w97 -> [_ _ w156]
                tunnel: w96 -> [_ _ w155]
                tunnel: w95 -> [_ _ w144]
                tunnel: w94 -> [w102 _ _]
                tunnel: w92 -> [w99 _ w143]
                tunnel: w91 -> [w98 _ _]
                tunnel: w90 -> [_ _ w140]
                tunnel: w89 -> [_ _ w138]
                frame #0 {
                  w111 = 1 items=["OneChannelForEachLine", "OneChannelForAllLines"] ("line grouping")
                  n75 = Decrement(x=w102) -> (x-1=w101:i32)
                  n76 = Multiply(x=8, y=w101) -> (x*y=w103:i32)
                  n77 = Add(x=w103, y=w99) -> (x+y=w100:i32)
                  n78 = Decrement(x=w98) -> (x-1=w112:dbl)
                  n79 = case shown="0, Default" w112 {
                    tunnel: [refnum<k21> "Dev0/1stPortA" ("Port 2") refnum<k21> "Dev0/1stPortB" ("Port 2") refnum<k21> "Dev1/1stPortA" ("Port 2") refnum<k21> "Dev1/1stPortB" ("Port 2")] -> w113
                    frame 0, Default {
                    }
                    frame 1 {
                    }
                    frame 2 {
                    }
                    frame 3 {
                    }
                  }
                  n80 = call-poly <vilib>:"ULx Create Virtual Channel.vi"("lines"=w113, "line grouping"=w111) -> ("task out"=w109:refnum<k24>, "error out"=w110:errorcluster)  [unwired: 12 in]
                  n81 = call <vilib>:"ULx Start Task.vi"("task in"=w109, "error in"=w110) -> ("task out"=w106:refnum<k24>, "error out"=w105:errorcluster)  [unwired: 12 in]
                  n82 = call-poly <vilib>:"ULx Write.vi"("task in"=w106, "data"=w100, "error in"=w105) -> ("task out"=w108:refnum<k24>, "error out"=w107:errorcluster)  [unwired: 10 in, 1 out]
                  n83 = call <vilib>:"ULx Clear Task.vi"("task in"=w108, "error in"=w107) -> ()  [unwired: 13 in, 1 out]
                }
                frame #1 {
                  n84 = Wait (ms)(milliseconds to wait=250) -> ()  [unwired: 1 out]
                }
                frame #2 {
                  n85 = Increment(x=w143) -> (x+1=w142:i32)
                  n86 = Index Array(array=w156, index=w155) -> (element=w141:T4)
                  n87 = Unbundle By Name(w141) -> ("Maximum Voltage (V)"=w145:dbl, "Minimum Voltage (V)"=w150:dbl, "Scan Direction\nDU (T), UD (F)"=w148:bool, "Step Size (V)"=w152:dbl, "Source Delay (s)"=w146:dbl)
                  n88 = Not(x=w148) -> (.not. x?=w149:bool)
                  n89 = Subtract(x=w145, y=w150) -> (x-y=w153:dbl)
                  n90 = Boolean To (0,1)(Boolean=w148) -> (0, 1=w147:i16)
                  n91 = Divide(x=w153, y=w152) -> (x/y=w154:dbl)
                  n92 = Boolean To (0,1)(Boolean=w149) -> (0, 1=w139:i16)
                  n93 = Increment(x=w154) -> (x+1=w151:dbl)
                  n94 = flat-sequence {
                    tunnel: "VISA resource name" -> [w172]
                    tunnel: w151 -> [w166]
                    tunnel: w150 -> [w167]
                    tunnel: w147 -> [w158]
                    tunnel: w146 -> [w159]
                    tunnel: w145 -> [w168]
                    tunnel: w144 -> [w162]
                    tunnel: w142 -> [w164]
                    tunnel: w141 -> [w161]
                    tunnel: w140 -> [w165]
                    tunnel: w138 -> [w160]
                    tunnel: w139 -> [w163]
                    tunnel: [w171] -> w137
                    tunnel: [w170] -> w136
                    tunnel: [w169] -> w135
                    tunnel: [w168] -> w134
                    tunnel: [w167] -> w133
                    tunnel: [w166] -> w132
                    tunnel: [w165] -> w131
                    tunnel: [w164] -> w130
                    tunnel: [w163] -> w129
                    tunnel: [w162] -> w128
                    tunnel: [w161] -> w127
                    tunnel: [w160] -> w126
                    tunnel: [w159] -> w125
                    tunnel: w137 -> [w180]
                    tunnel: w136 -> [w177]
                    tunnel: w135 -> [w188]
                    tunnel: w134 -> [w189]
                    tunnel: w133 -> [w187]
                    tunnel: w132 -> [w186]
                    tunnel: w131 -> [w185]
                    tunnel: w130 -> [w184]
                    tunnel: w129 -> [w173]
                    tunnel: w128 -> [w183]
                    tunnel: w127 -> [w182]
                    tunnel: w126 -> [w181]
                    tunnel: w125 -> [w179]
                    tunnel: [w178] -> w124
                    tunnel: [w177] -> w123
                    tunnel: [w176] -> w122
                    tunnel: [w175] -> w121
                    tunnel: [w174] -> w120
                    tunnel: w124 -> [w190]
                    tunnel: w123 -> [w197]
                    tunnel: w122 -> [w196]
                    tunnel: w121 -> [w195]
                    tunnel: w120 -> [w191]
                    tunnel: [w190] -> w119
                    tunnel: w119 -> [w200]
                    frame #0 {
                      n95 = call "Keithley Sweep and Acquire Measurements.vi"("Source Delay (s)"=w159, "Sweep Direction"=w158, "Number of Points"=w166, "Maximum Amplitude"=w168, "Minimum Amplitude"=w167, "VISA resource name"=w172) -> ("Data Array"=w170:dbl[][], "VISA resource name out"=w171:refnum<visa-resource-name>)  [unwired: 1 in, 1 out]
                      n96 = local read "Username"() -> (w169:string)
                      n97 = call "Save Data.vi"("Experiment Indicator"=w165, "Username"=w169, "Pixel"=w164, "Scan direction"=w158, "Data Array"=w170, "Cell details cluster"=w162, "Show me Scan \nSettings JV set"=w161, "Time zero"=w160) -> ()  [unwired: 3 in, 5 out]
                    }
                    frame #1 {
                      n98 = call "Keithley Sweep and Acquire Measurements.vi"("Source Delay (s)"=w179, "Sweep Direction"=w173, "Number of Points"=w186, "Maximum Amplitude"=w189, "Minimum Amplitude"=w187, "VISA resource name"=w180) -> ("Data Array"=w176:dbl[][], "VISA resource name out"=w174:refnum<visa-resource-name>)  [unwired: 1 in, 1 out]
                      n99 = call "Save Data.vi"("Experiment Indicator"=w185, "Username"=w188, "Pixel"=w184, "Scan direction"=w173, "Data Array"=w176, "Cell details cluster"=w183, "Show me Scan \nSettings JV set"=w182, "Time zero"=w181) -> ("Master Log"=w175:string[][], "File path for JV image"=w178:path)  [unwired: 3 in, 3 out]
                    }
                    frame #2 {
                      n100 = call "Format data to plot.vi"("Data Array 2"=w196, "Data Array"=w197) -> ("JV Curve"=→"JV Curve":cluster{"Y":dbl[], "Y":dbl[]}[])  [unwired: 9 in]
                      n101 = call <instrlib>:"Enable Output.vi"("Enable Output (T: Enable)"=FALSE, "VISA resource name"=w191) -> ("error out"=w193:errorcluster, "VISA resource name out"=w194:refnum<visa-resource-name>)  [unwired: 8 in]
                      n102 = invoke on="JV Curve" class="XYGraph (strict)" method="Get Image"() -> ("image data"=w199:T9)  [unwired: 6 in, 5 out]
                      n103 = call <instrlib>:"Close.vi"("error in (no error)"=w193, "VISA resource name"=w194) -> ()  [unwired: 9 in, 1 out]
                      n104 = call <vilib>:"Write JPEG File.vi"("image data"=w199, "path to JPEG file"=w190) -> ()  [unwired: 8 in, 2 out]
                      "Table" <- w195
                    }
                    frame #3 {
                      n105 = call "Copy file to network and group server.vi"("File path in"=w200) -> ()  [unwired: 11 in]
                    }
                  }
                }
              }
              n106 = Equal?(x=7, y=w92) -> (x = y?=w88:bool)
            }
            n107 = Compound Arithmetic op=OR(w81, "Stop Scan") -> (w84:bool)
          }
        }
      }
    }
    n108 = Index Array(array=w11, index="Scan settings") -> (element=→"Show me Scan \nSettings JV set":T4)
    n109 = case shown="True" "Save to Spreadsheet?  3" {
      frame False {
      }
      frame True {
        n110 = local read "Cell Settings Array 3"() -> (w49:T1)
        n111 = call "save_to_file.vi"("Cell Settings Array 4"=w49, "Save Path"="Save Spreadsheet Path 3") -> ()  [unwired: 1 in]
      }
    }
    n112 = case shown="True" "Upload from Spreadsheet? 3" {
      frame False {
      }
      frame True {
        n113 = call "upload_from_file.vi"("Spreadsheet path"="Upload Spreadsheet path 3") -> ("Cell Settings Array 4"=w51:T1)
        n114 = local write "Cell Settings Array 3"(w51) -> ()
      }
    }
    n115 = case shown="False" "Save to Spreadsheet?  4" {
      frame False {
      }
      frame True {
        n116 = local read "Cell Settings Array 4"() -> (w45:T1)
        n117 = call "save_to_file.vi"("Cell Settings Array 4"=w45, "Save Path"="Save Spreadsheet Path 4") -> ()  [unwired: 1 in]
      }
    }
    n118 = case shown="True" "Upload from Spreadsheet? 4" {
      frame False {
      }
      frame True {
        n119 = call "upload_from_file.vi"("Spreadsheet path"="Upload Spreadsheet path 4") -> ("Cell Settings Array 4"=w47:T1)
        n120 = local write "Cell Settings Array 4"(w47) -> ()
      }
    }
    n121 = local write "Queue"(w9) -> ()
  }
